vi "RGRFinal.vi"() -> ()   [LabVIEW 2014]
uses:
  <vilib>/Instr/_visa.llb/VISA Configure Serial Port (Instr).vi
  <vilib>/Utility/file.llb/Read From Spreadsheet File (string).vi
  <vilib>/Utility/file.llb/Write To Spreadsheet File (string).vi
  <vilib>/express/express arith-compare/Formula/XNode/ExpressFormulaBlockNode.xnode
panel:
  out "Waveform Graph":dbl[](graph)
  out "Table Control":string[][](table)
  in  "file path (dialog if empty)":path
  out "Arduino Data":i32
  out "Voltage":dbl format="%#_3g"
  out "Percent":dbl format="%#_3g"
  in  "VISA resource name":refnum<visa-resource-name>
  in  "baud rate (9600)":u32=9600
  out "error out":errorcluster
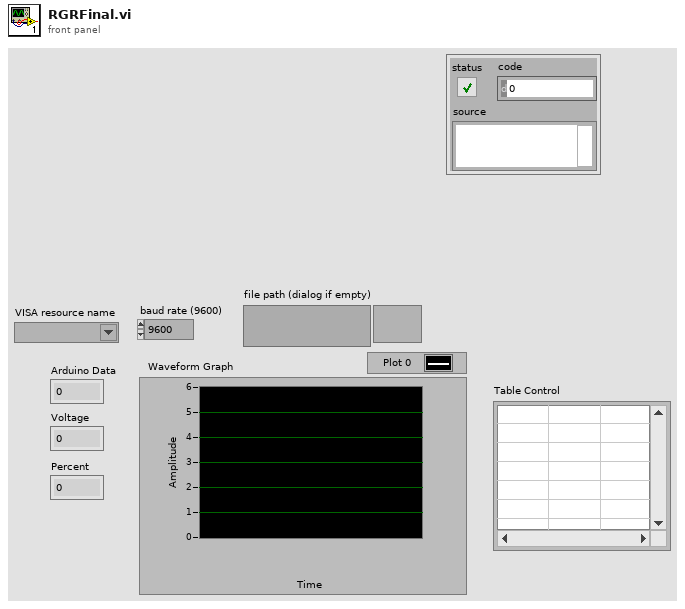
[diagram p1: front panel]
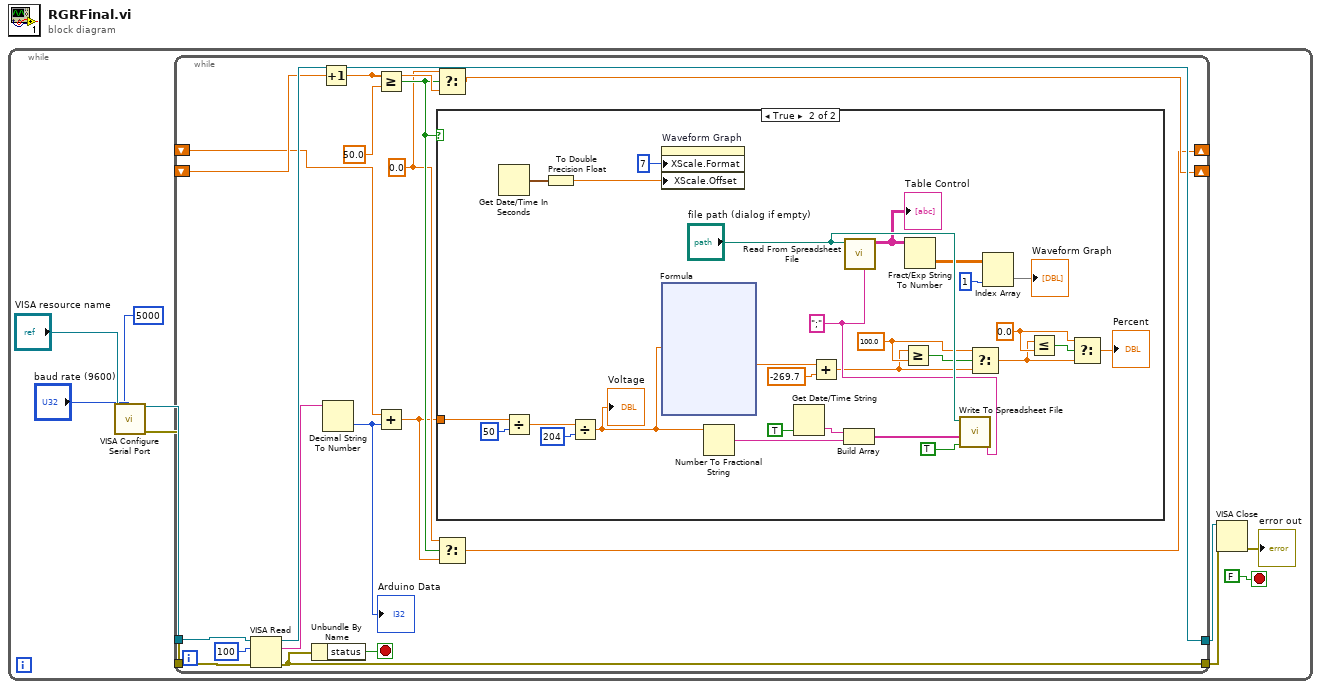
[diagram p0: block diagram]
diagram:
  n1 = while {
    stop <- FALSE stop-if-true
    n2 = call-poly "VISA Configure Serial Port"("VISA resource name"="VISA resource name", "timeout (10sec)"=u32 5000, "baud rate (9600)"="baud rate (9600)") -> ("VISA resource name out"=w9:refnum<visa-resource-name>, "error out"=w8:errorcluster)  [unwired: 11 in]
    n3 = while {
      tunnel: w9 -> [w26]
      tunnel: w8 -> [w23]
      tunnel: [w18] -> w7
      tunnel: [w25] -> w6
      shift-right: [w20] -> _
      shift-left: _ -> [w22]
      shift-right: [w12] -> _
      shift-left: _ -> [w11]
      stop <- w17 stop-if-true
      w15 = 0.0 ("t")
      n4 = VISA Read(VISA resource name=w26, byte count=u32 100, error in (no error)=w23) -> (VISA resource name out=w25:refnum<visa-resource-name>, read buffer=w19:string, error out=w18:errorcluster)  [unwired: 1 out]
      n5 = Unbundle By Name(w18) -> ("status"=w17:bool)
      n6 = Increment(x=w22) -> (x+1=w21:dbl)
      n7 = Decimal String To Number(string=w19) -> (number=w13:i32)  [unwired: 2 in, 1 out]
      "Arduino Data" <- w13
      n8 = Greater Or Equal?(x=w21, y=50.0) -> (x >= y?=w16:bool)
      n9 = Add(x=w11, y=w13) -> (x+y=w10:dbl)
      n10 = Select(t=w15, s=w16, f=w21) -> (s? t:f=w20:dbl)
      n11 = case shown="True" w16 {
        tunnel: w10 -> [_ w38]
        frame False {
        }
        frame True {
          w29 = 0.0 ("y")
          w32 = 100.0 ("y")
          w50 = ";" ("delimiter (\\t)")
          n12 = Get Date/Time In Seconds() -> (seconds since 1Jan1904=w41:timestamp)
          n13 = Divide(x=w38, y=50) -> (x/y=w37:dbl)
          n14 = To Double Precision Float(number=w41) -> (double precision float=w40:dbl)
          n15 = Divide(x=w37, y=204) -> (x/y=w35:dbl)
          "Voltage" <- w35
          n16 = property on="Waveform Graph" class="WFGraph (strict)"("XScale.Format"=u8 7 ("X Scale.Display Format:Format"), "XScale.Offset"=w40) -> ()  [unwired: 2 in, 2 out]
          n17 = xnode "Formula"("m"=w35) -> ("Result"=w34:dbl)  [unwired: 1 in, 1 out]
          n18 = Number To Fractional String(number=w35) -> (F-format string=w49:string)  [unwired: 3 in]
          n19 = Get Date/Time String(want seconds? (F)=TRUE) -> (time string=w48:string)  [unwired: 2 in, 1 out]
          n20 = Add(x=w34, y=-269.7) -> (x+y=w31:dbl)
          n21 = Build Array(w48, w49) -> (w52:string[])
          n22 = call-poly <vilib>:"Read From Spreadsheet File.vi"("delimiter (\\t)"=w50, "file path (dialog if empty)"="file path (dialog if empty)") -> ("all rows"=w46:string[][])  [unwired: 5 in, 4 out]
          "Table Control" <- w46
          n23 = Greater Or Equal?(x=w31, y=w32) -> (x >= y?=w33:bool)
          n24 = Fract/Exp String To Number(string=w46) -> (number=w45:dbl[][])  [unwired: 3 in, 1 out]
          n25 = call-poly <vilib>:"Write To Spreadsheet File.vi"("delimiter (\\t)"=w50, "append to file? (new file:F)"=TRUE, "1D data"=w52, "file path (dialog if empty)"="file path (dialog if empty)") -> ()  [unwired: 4 in, 1 out]
          n26 = Select(t=w32, s=w33, f=w31) -> (s? t:f=w28:dbl)
          n27 = Index Array(array=w45, index (col)=1 ("disabled index (col)")) -> (element=→"Waveform Graph":dbl[])  [unwired: 1 in]
          n28 = Less Or Equal?(x=w28, y=w29) -> (x <= y?=w30:bool)
          n29 = Select(t=w29, s=w30, f=w28) -> (s? t:f=→"Percent":dbl)
        }
      }
      n30 = Select(t=w15, s=w16, f=w10) -> (s? t:f=w12:dbl)
    }
    n31 = VISA Close(VISA resource name=w6, error in (no error)=w7) -> (error out=→"error out":errorcluster)
  }
